vi "theNarrator.vi"(11 "IA state":T1={"our_robots"=[], "enemy_robots"=[], "balls"=[], "geometry"={"line_width"=0, "field_length"=0, "field_width"=0, "boundary_width"=0, "referee_width"=0, "goal_width"=0, "goal_depth"=0, "goal_wall_width"=0, "center_circle_radius"=0, "defense_radius"=0, "defense_stretch"=0, "free_kick_from_defense_dist"=0, "penalty_spot_from_field_line_dist"=0, "penalty_line_from_spot_dist"=0}, "IA Judge"={"stage"="", "command"="", "our_goalie_id"=0.0, "enemy_goalie_id"=0.0, "command enum"=enum."Halt", "Time"=enum."Azul"}, "Received Timestamp"=timestamp(0 s since 1904-01-01), "Events"={"Touch"=FALSE, "Ball out"=FALSE, "id touch"=0.0, "Ball out of \nVision"=FALSE, "Ball inside \nGoalie area"=FALSE, "Robot not responding"=FALSE, "Robots responding status"=[1.0, 1.0, 1.0, 1.0, 1.0, 1.0], "Enemy Ball \nPossession"=FALSE, "Pass State"=FALSE, "id end of pass"=0.0, "Kick"=FALSE, "Id ini Possession"=0.0, "Ball Possesion"=FALSE, "Id Possesion"=0.0}}) -> ()   [LabVIEW 2017]
uses:
  Core/AI Input.ctl
  Core/AI Robot.ctl
  Intel/Functions Enum.ctl
  Intel/AttackerStates.ctl
  Core/AI Ball.ctl
  Core/Field Size.ctl
  Core/AI Judge.ctl
  Intel/Command Enum.ctl
  Util/Events/Events.ctl
panel:
  in  "Linhas exibidas":i32=4
  out "Ultimas linhas":string[](array[string])
  out "concatenated string":string
  out "error out":errorcluster
  out "path out":path
  in  "error in":errorcluster
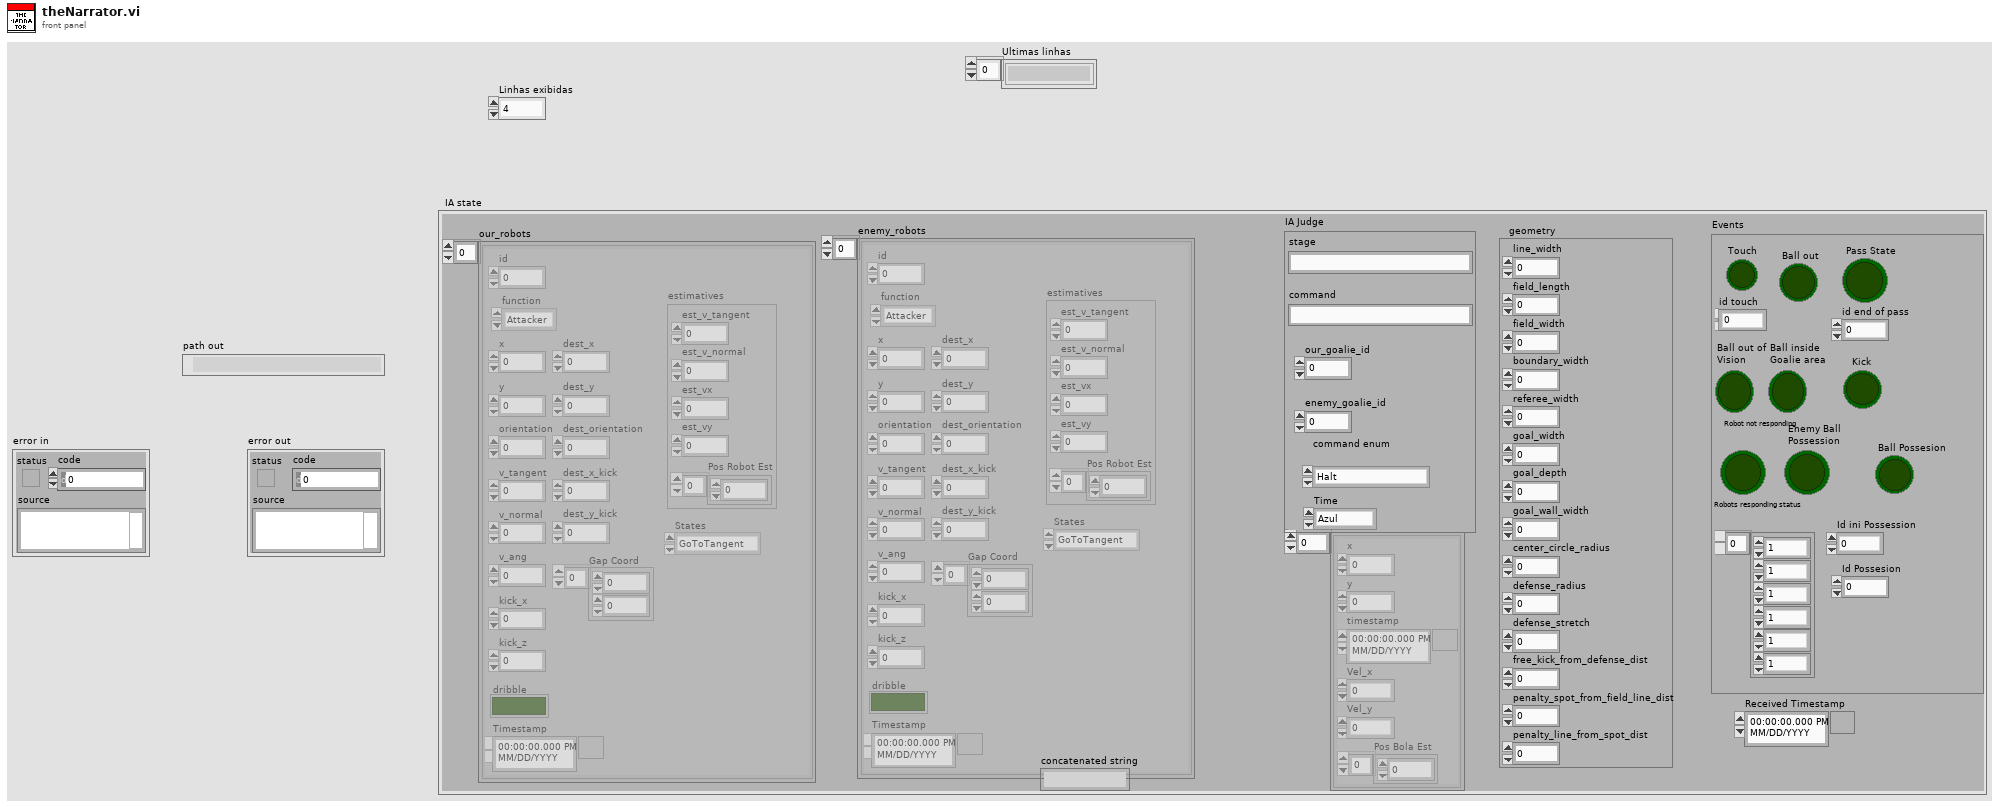
[diagram p1: front panel]
types:
  T1 = typedef "AI Input.ctl" = cluster{"our_robots":T2[], "enemy_robots":T2[], "balls":T5[], "geometry":T6, "IA Judge":T7, "Received Timestamp":timestamp, "Events":T9}
  T2 = typedef "AI Robot.ctl" = cluster{"id":u32, "function":T3, "x":dbl, "y":dbl, "orientation":dbl, "v_tangent":dbl, "v_normal":dbl, "v_ang":dbl, "kick_x":dbl, "kick_z":dbl, "dribble":bool, "Timestamp":timestamp, "dest_x":dbl, "dest_y":dbl, "dest_orientation":dbl, "estimatives":cluster{"est_v_tangent":dbl, "est_v_normal":dbl, "est_vx":dbl, "est_vy":dbl, "Pos Robot Est":dbl[]}, "dest_x_kick":dbl, "dest_y_kick":dbl, "Gap Coord":dbl[], "States":T4}
  T3 = typedef "Functions Enum.ctl" = enum16{"Attacker", "Goalie", "Defender", "Striker", "Goto 0", "Dummy", "Kicker", "ZigZag"}
  T4 = typedef "AttackerStates.ctl" = enum16{"Pass", "GoToTangent", "BallGetting", "GoToKick", ""}
  T5 = typedef "AI Ball.ctl" = cluster{"x":dbl, "y":dbl, "timestamp":timestamp, "Vel_x":dbl, "Vel_y":dbl, "Pos Bola Est":dbl[]}
  T6 = typedef "Field Size.ctl" = cluster{"line_width":u32, "field_length":u32, "field_width":u32, "boundary_width":u32, "referee_width":u32, "goal_width":u32, "goal_depth":u32, "goal_wall_width":u32, "center_circle_radius":u32, "defense_radius":u32, "defense_stretch":u32, "free_kick_from_defense_dist":u32, "penalty_spot_from_field_line_dist":u32, "penalty_line_from_spot_dist":u32}
  T7 = typedef "AI Judge.ctl" = cluster{"stage":string, "command":string, "our_goalie_id":dbl, "enemy_goalie_id":dbl, "command enum":T8, "Time":enum16{"Azul", "Amarelo"}}
  T8 = typedef "Command Enum.ctl" = enum16{"Halt", "Stop", "Force Start", "PKA Normal Start", "Prepare Kickoff Ally", "PKE Normal Start", "Prepare Kickoff Enemy", "Prepare Penalty Ally", "PPA Normal Start", "Prepare Penalty Enemy", "PPE Normal Start", "Direct Free Enemy", "Direct Free Ally", "Indirect Free Enemy", "Indirect Free Ally", "Timeout Enemy", "Timeout Ally", "Goal Enemy", "Goal Ally", "Ball Placement Enemy", "Ball Placement Ally", "Normal Half Time", "Extra Time Break", "Extra Half Time", "None", "Post Game"}
  T9 = typedef "Events.ctl" = cluster{"Touch":bool, "Ball out":bool, "id touch":dbl, "Ball out of \nVision":bool, "Ball inside \nGoalie area":bool, "Robot not responding":bool, "Robots responding status":dbl[], "Enemy Ball \nPossession":bool, "Pass State":bool, "id end of pass":dbl, "Kick":bool, "Id ini Possession":dbl, "Ball Possesion":bool, "Id Possesion":dbl}
  T10 = enum16{"open", "replace", "create", "open or create", "replace or create", "replace or create with confirmation"}
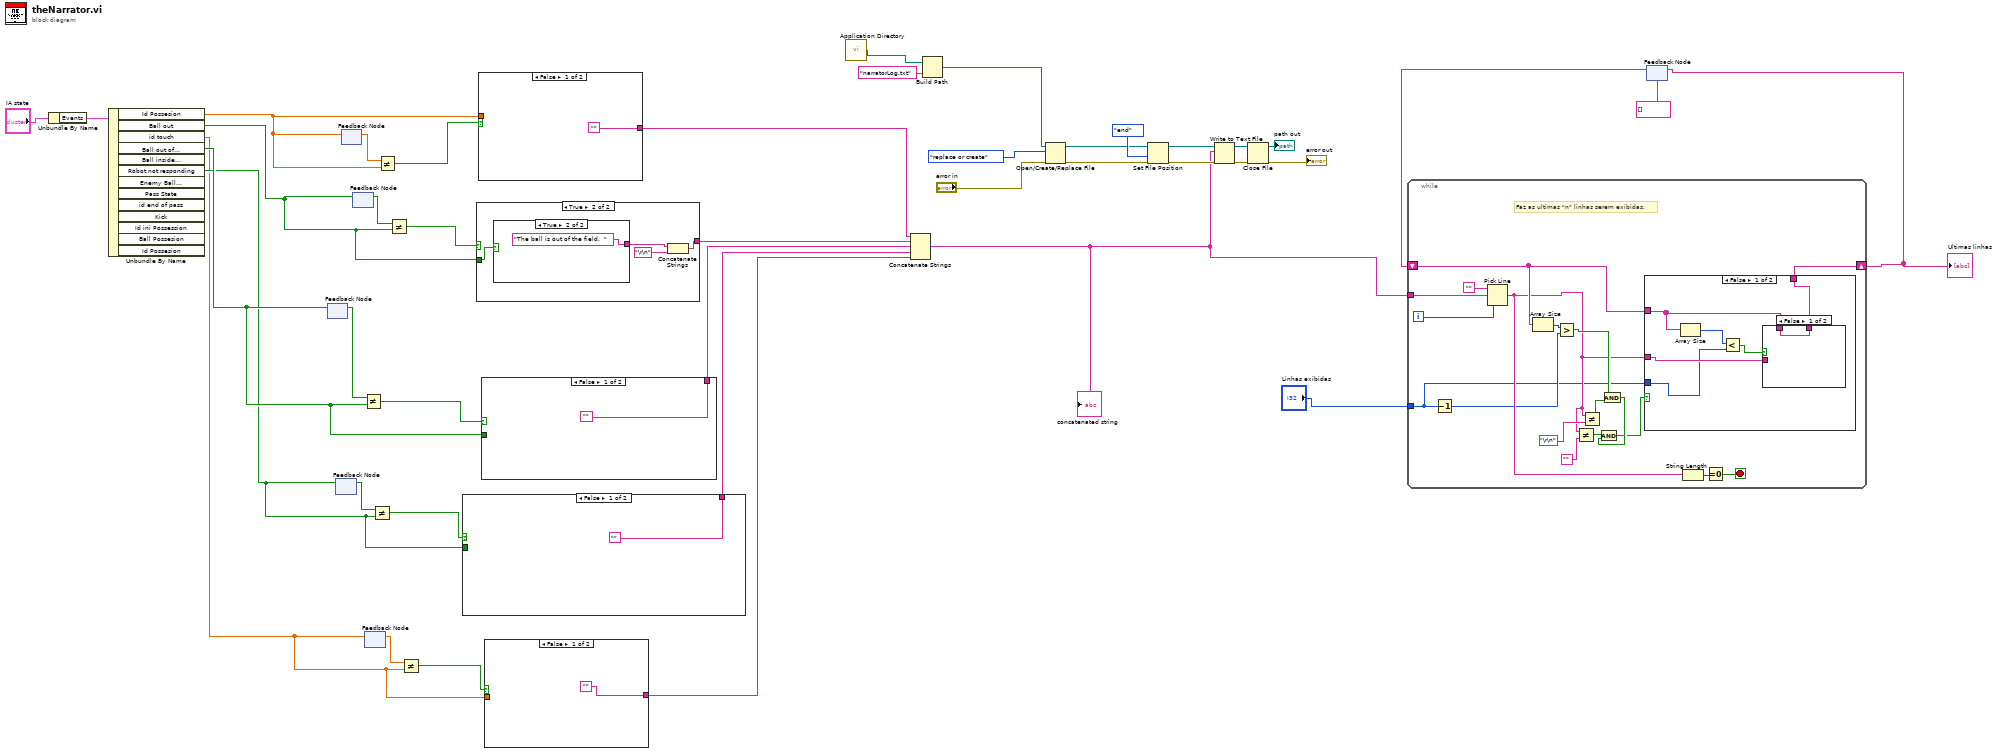
[diagram p0: block diagram]
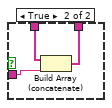
[diagram p2: hidden frame]
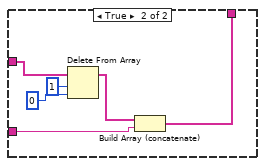
[diagram p3: hidden frame]
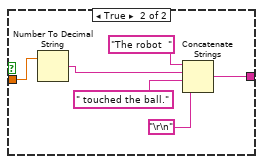
[diagram p4: hidden frame]
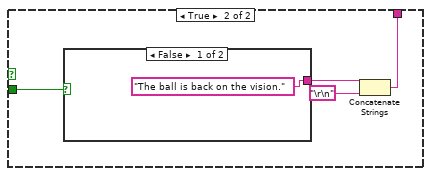
[diagram p5: hidden frame]
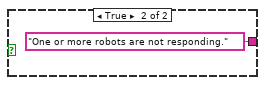
[diagram p6: hidden frame]
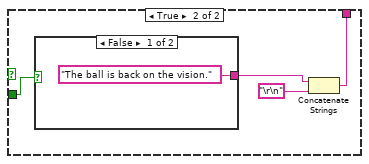
[diagram p7: hidden frame]
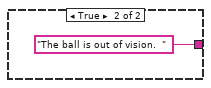
[diagram p8: hidden frame]
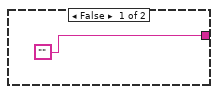
[diagram p9: hidden frame]
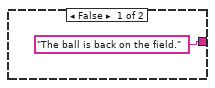
[diagram p10: hidden frame]
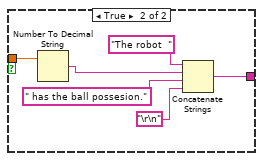
[diagram p11: hidden frame]
diagram:
  n1 = Unbundle By Name("IA state") -> ("Events"=w29:T9)
  n2 = Unbundle By Name(w29) -> ("Id Possesion"=w28:dbl, "Ball out"=w23:bool, "id touch"=w14:dbl, "Ball out of \nVision"=w21:bool, "Robot not responding"=w17:bool)  [unwired: 8 out]
  n3 = feedback #1() -> (w22:bool)  [unwired: 1 in]
  n4 = feedback-in #1(w21) -> ()
  n5 = feedback #2() -> (w19:bool)  [unwired: 1 in]
  n6 = feedback-in #2(w17) -> ()
  n7 = feedback-in #3(w28) -> ()
  n8 = feedback #3() -> (w27:dbl)  [unwired: 1 in]
  n9 = feedback #4() -> (w26:bool)  [unwired: 1 in]
  n10 = feedback-in #4(w23) -> ()
  n11 = Not Equal?(x=w22, y=w21) -> (x != y?=w20:bool)
  n12 = feedback #5() -> (w16:dbl)  [unwired: 1 in]
  n13 = feedback-in #5(w14) -> ()
  n14 = Not Equal?(x=w19, y=w17) -> (x != y?=w18:bool)
  n15 = Not Equal?(x=w27, y=w28) -> (x != y?=w25:bool)
  n16 = Not Equal?(x=w26, y=w23) -> (x != y?=w24:bool)
  n17 = Not Equal?(x=w16, y=w14) -> (x != y?=w15:bool)
  n18 = case shown="False" w18 {
    tunnel: w17 -> [_ w46]
    tunnel: ["" w43] -> w10
    frame False {
    }
    frame True {
      n19 = case shown="False" w46 {
        tunnel: ["The ball is back on the vision." ("string") "One or more robots are not responding." ("string")] -> w44
        frame False {
        }
        frame True {
        }
      }
      n20 = Concatenate Strings(w44, "\r\n") -> (w43:string)
    }
  }
  n21 = case shown="True" w24 {
    tunnel: w23 -> [_ w53]
    tunnel: ["" w50] -> w12
    frame False {
    }
    frame True {
      n22 = case shown="True" w53 {
        tunnel: ["The ball is back on the field." ("string") "The ball is out of the field.  " ("string")] -> w51
        frame False {
        }
        frame True {
        }
      }
      n23 = Concatenate Strings(w51, "\r\n") -> (w50:string)
    }
  }
  n24 = case shown="False" w25 {
    tunnel: w28 -> [_ w59]
    tunnel: ["" w57] -> w13
    frame False {
    }
    frame True {
      n25 = Number To Decimal String(number=w59) -> (decimal integer string=w61:string)  [unwired: 1 in]
      n26 = Concatenate Strings("The robot  " ("string"), w61, " has the ball possesion." ("string"), "\r\n") -> (w57:string)
    }
  }
  n27 = case shown="False" w20 {
    tunnel: w21 -> [_ w67]
    tunnel: ["" w64] -> w11
    frame False {
    }
    frame True {
      n28 = case shown="False" w67 {
        tunnel: ["The ball is back on the vision." ("string") "The ball is out of vision.  " ("string")] -> w65
        frame False {
        }
        frame True {
        }
      }
      n29 = Concatenate Strings(w65, "\r\n") -> (w64:string)
    }
  }
  n30 = case shown="False" w15 {
    tunnel: w14 -> [_ w73]
    tunnel: ["" w71] -> w9
    frame False {
    }
    frame True {
      n31 = Number To Decimal String(number=w73) -> (decimal integer string=w75:string)  [unwired: 1 in]
      n32 = Concatenate Strings("The robot  " ("string"), w75, " touched the ball." ("string"), "\r\n") -> (w71:string)
    }
  }
  n33 = call <vilib>:"Application Directory.vi"() -> ("Application Directory"=w6:path)
  n34 = Concatenate Strings(w13, w12, w11, w10, w9) -> (w5:string)
  "concatenated string" <- w5
  n35 = Build Path(base path=w6, name or relative path="narratorLog.txt") -> (appended path=w7:path)
  n36 = Open/Create/Replace File(file path (use dialog)=w7, error in="error in", operation (0:open)=T10."replace or create") -> (refnum out=w36:refnum<file>, error out=w37:errorcluster)  [unwired: 3 in, 1 out]
  n37 = Set File Position(refnum=w36, from (0:start)=enum16{"start", "end", "current"}."end", error in=w37) -> (refnum out=w35:refnum<file>, error out=w34:errorcluster)  [unwired: 1 in]
  n38 = Write to Text File(file (use dialog)=w35, text=w5, error in=w34) -> (refnum out=w41:refnum<file>, error out=w40:errorcluster)  [unwired: 1 in, 1 out]
  n39 = Close File(refnum=w41, error in=w40) -> (path=→"path out":path, error out=→"error out":errorcluster)
  n40 = feedback #6(string[] []) -> (w4:string[])
  n41 = while {
    shift-right: [w84] -> w3
    shift-left: w4 -> [w88]
    tunnel: w5 -> [w90]
    tunnel: "Linhas exibidas" -> [w77]
    i -> [w94]
    stop <- w91 stop-if-true
    # "Faz as ultimas \"n\" linhas serem exibidas."
    n42 = Decrement(x=w77) -> (x-1=w78:i32)
    n43 = Pick Line(string ("")="", multi-line string=w90, line index=w94) -> (output string=w81:string)
    n44 = Array Size(array=w88) -> (size(s)=w89:i32)
    n45 = Greater?(x=w89, y=w78) -> (0:w87:bool)
    n46 = Not Equal?(x=w81, y="") -> (x != y?=w83:bool)
    n47 = Not Equal?(x=w81, y="\r\n") -> (x != y?=w86:bool)
    n48 = And(x=w87, y=w86) -> (x .and. y?=w80:bool)
    n49 = And(x=w83, y=w80) -> (x .and. y?=w79:bool)
    n50 = case shown="False" w79 {
      tunnel: w88 -> [w98 w108]
      tunnel: [w96 w109] -> w84
      tunnel: w81 -> [w97 w110]
      tunnel: w77 -> [w95 _]
      frame False {
        n51 = Array Size(array=w98) -> (size(s)=w100:i32)
        n52 = Less?(x=w100, y=w95) -> (x < y?=w99:bool)
        n53 = case shown="False" w99 {
          tunnel: w98 -> [w101 w104]
          tunnel: w97 -> [_ w103]
          tunnel: [w101 w102] -> w96
          frame False {
          }
          frame True {
            n54 = Build Array (concatenate)(w104, w103) -> (w102:string[])
          }
        }
      }
      frame True {
        n55 = Delete From Array(array=w108, length=1, index=0) -> (array with subset deleted=w105:string[])  [unwired: 1 out]
        n56 = Build Array (concatenate)(w105, w110) -> (w109:string[])
      }
    }
    n57 = String Length(string=w81) -> (length=w92:i32)
    n58 = Equal To 0?(x=w92) -> (x = 0?=w91:bool)
  }
  "Ultimas linhas" <- w3
  n59 = feedback-in #6(w3) -> ()
